vi "test_Switch Scalar Type to Bitpacked Type.vi"(8 "error in (no error)":errorcluster, 11 "TestCase in":refnum<class "Scalar Bitpacking Testing.lvclass">) -> (0 "error out":errorcluster, 3 "TestCase out":refnum<class "Scalar Bitpacking Testing.lvclass">)   [LabVIEW 2019, in "Scalar Bitpacking Testing.lvclass"]
uses:
  Scalar Bitpacking Testing.lvclass
  Scalar Bitpacking Testing.lvclass/Scalar Bitpacking Testing.ctl
  Addon/Addon Shared/SubVIs/Constants.vi
  <vilib>/NI/NI VeriStand Advanced SysDef API/_SubVIs/SysDef.Search.GUID.vi
  <vilib>/NI/NI VeriStand Advanced SysDef API/_SubVIs/SysDef.Search.GUIDs.vi
  <vilib>/addons/_JKI Toolkits/VI Tester/TestCase.llb/TestCase.lvclass
  Addon/Addon System Explorer/FPGA Addon System Explorer.lvlib
  <vilib>/NI/NI VeriStand Advanced SysDef API/SysDef API/Advanced System Definition.lvlib
  Addon/Addon Shared/FPGA Addon Shared.lvlib
  C:/Program Files (x86)/National Instruments/LabVIEW 2019/vi.lib/addons/_JKI Toolkits/VI Tester/TestCase.llb/TestCase.lvclass
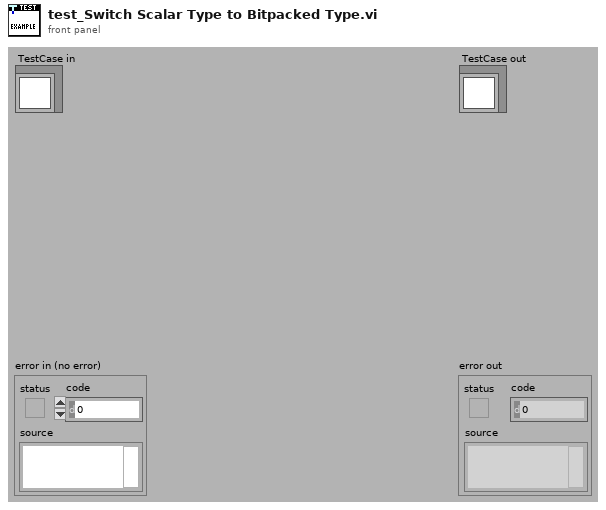
[diagram p1: front panel]
types:
  T1 = typedef "Advanced System Definition.lvlib/TreeItem.Info.ctl" = cluster{"Name":string, "Description":string, "GUID":string, "Is Channel":bool, "Channel":T2, "Is Waveform":bool, "Waveform":T4}
  T2 = typedef "Custom Device API.lvlib/Custom Device Channel.ctl" = cluster{"Type":T3, "Units":string, "Default Value":dbl, "Faultable":bool, "Scalable":bool}
  T3 = typedef "Custom Device API.lvlib/Custom Device Channel Type.ctl" = enum16{"Input", "Output"}
  T4 = typedef "Custom Device API.lvlib/Custom Device Waveform.ctl" = cluster{"Data Type":T5, "Units":string}
  T5 = typedef "Custom Device API.lvlib/Custom Device Waveform DataType.ctl" = enum16{"Double", "Complex Double"}
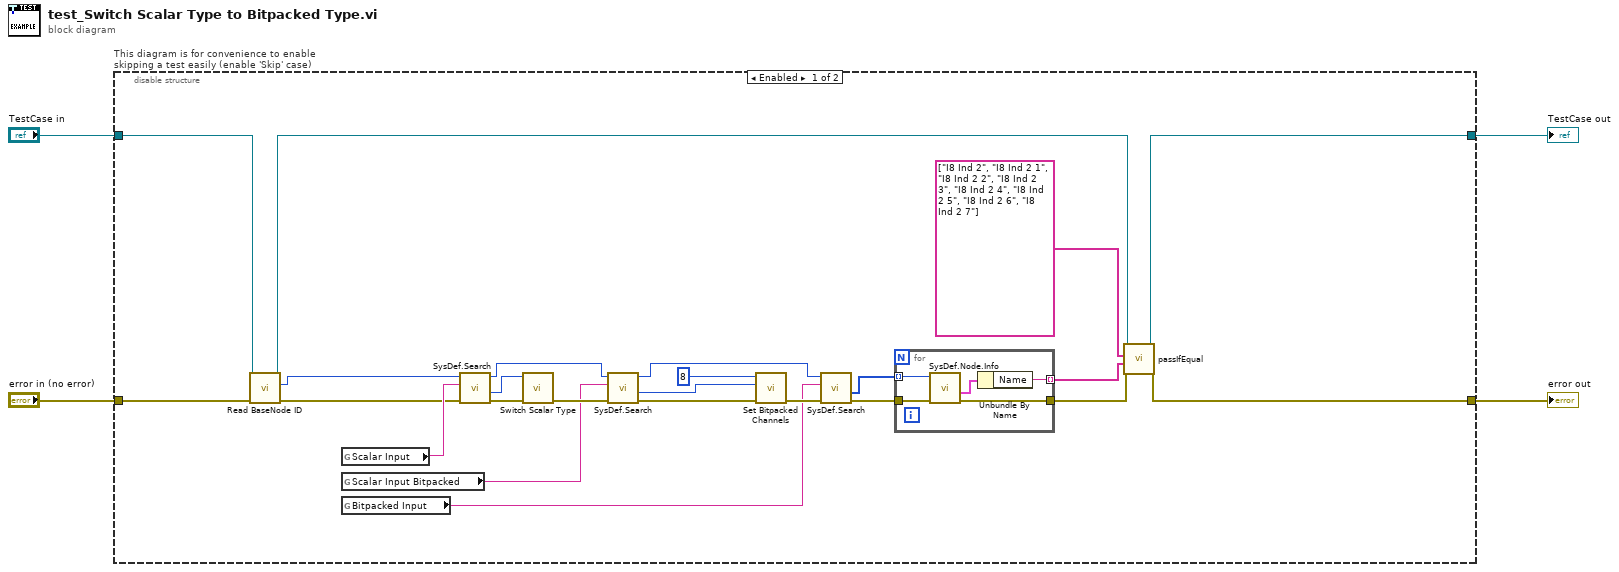
[diagram p0: block diagram]
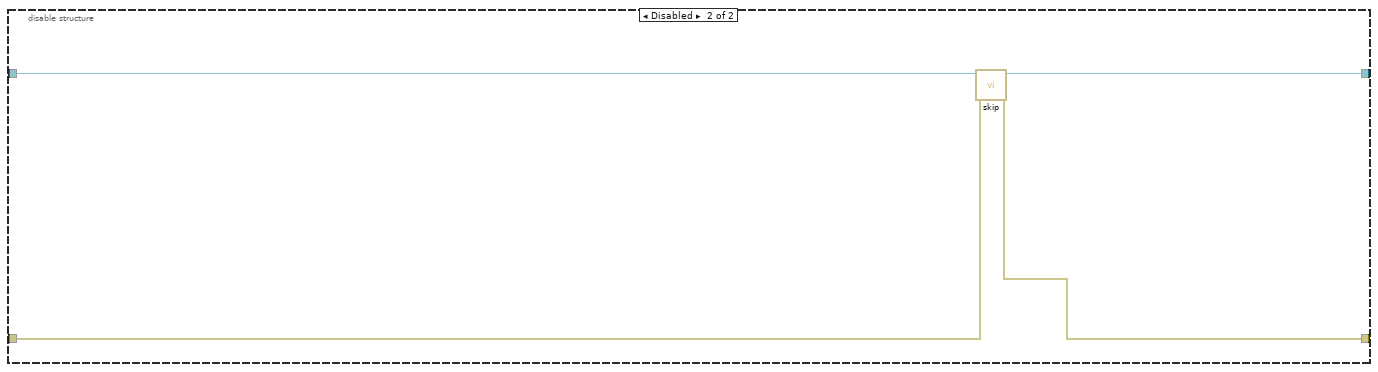
[diagram p2: hidden frame]
diagram:
  n1 = disable-structure "This diagram is for convenience to enable skipping a test easily (enable 'Skip' case)" shown="Enabled" {
    disable-tunnel: "TestCase in" -> [w9 w37]
    disable-tunnel: [w28 w35] -> w1
    disable-tunnel: [w23 w36] -> w3
    disable-tunnel: "error in (no error)" -> [w8 w34]
    frame Enabled {
      n2 = call "Read BaseNode ID.vi"("error in (no error)"=w8, "Scalar Bitpacking Testing in"=w9) -> ("error out"=w7:errorcluster, "BaseNode ID"=w6:u64, "Scalar Bitpacking Testing out"=w5:refnum<class "Scalar Bitpacking Testing.lvclass">)  [unwired: 7 in]
      n3 = global read "Constants.vi" "Scalar Input"() -> (w15:string)
      n4 = global read "Constants.vi" "Scalar Input Bitpacked"() -> (w13:string)
      n5 = global read "Constants.vi" "Bitpacked Input"() -> (w12:string)
      n6 = call-poly <vilib>:"SysDef.Search.vi"("error in (no error)"=w7, "GUID"=w15, "nodeID"=w6) -> ("error out"=w21:errorcluster, "Value out"=w20:u64, "nodeID out"=w14:u64)  [unwired: 5 in, 1 out]
      n7 = call "Switch Scalar Type.vi"("error in (no error)"=w21, "Node Ptr"=w20) -> ("error out"=w19:errorcluster)  [unwired: 9 in]
      n8 = call-poly <vilib>:"SysDef.Search.vi"("error in (no error)"=w19, "GUID"=w13, "nodeID"=w14) -> ("error out"=w18:errorcluster, "Value out"=w17:u64, "nodeID out"=w16:u64)  [unwired: 5 in, 1 out]
      n9 = call "Set Bitpacked Channels.vi"("error in (no error)"=w18, "Item Ref in"=w17, "Number of Channels"=u8 8) -> ("error out"=w26:errorcluster)  [unwired: 8 in]
      n10 = call-poly <vilib>:"SysDef.Search.vi"("error in (no error)"=w26, "GUID"=w12, "nodeID"=w16) -> ("error out"=w24:errorcluster, "Values Out"=w25:u64[])  [unwired: 5 in, 2 out]
      n11 = for {
        tunnel: w25 -> [w33] mode=indexing
        tunnel: w24 -> [w31]
        tunnel: [w30] -> w22
        tunnel: [w29] -> w10 mode=indexing
        n12 = call <vilib>:"SysDef.Node.Info.vi"("error in (no error)"=w31, "nodeID"=w33) -> ("error out"=w30:errorcluster, "Item Info"=w32:T1)  [unwired: 6 in, 2 out]
        n13 = Unbundle By Name(w32) -> ("Name"=w29:string)
      }
      n14 = call-dynamic "passIfEqual.vi"("error in (no error)"=w22, "y"=w10, "x"=string[] ["I8 Ind 2", "I8 Ind 2 1", "I8 Ind 2 2", "I8 Ind 2 3", "I8 Ind 2 4", "I8 Ind 2 5", "I8 Ind 2 6", "I8 Ind 2 7"] ("Array"), "TestCase in"=w5) -> ("error out"=w23:errorcluster, "TestCase out"=w28:refnum<class "Scalar Bitpacking Testing.lvclass">)  [unwired: 6 in]
    }
    frame Disabled {
      # "skip test result while test is under development"
      n15 = call <vilib>:"skip.vi"("error in (no error)"=w34, "TestCase in"=w37) -> ("error out"=w36:errorcluster, "TestCase out"=w35:refnum<class "Scalar Bitpacking Testing.lvclass">)  [unwired: 8 in]
    }
  }
  "error out" <- w3
  "TestCase out" <- w1
